vi "OutputVoltage.vi"(8 "error in":errorcluster caption="错误输入（无错误）", 9 "Channel":i32(ring)=1 items=["Channel 1"=1, "Channel 2"=2], 10 "Voltage Level":dbl format="%.3g", 11 "VISAin":refnum<visa-resource-name>) -> (0 "error out":errorcluster caption="错误输出", 1 "time":u32, 3 "VISAout":refnum<visa-resource-name>)   [LabVIEW 2013]
panel:
  out "字符串":string
  out "结果字符串":string
  in  "Current Level":dbl=0.02 format="%.3g"
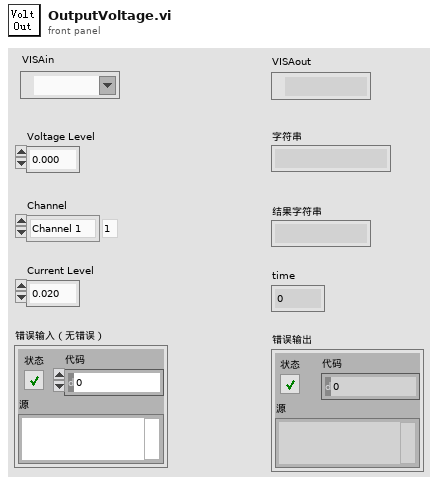
[diagram p1: front panel]
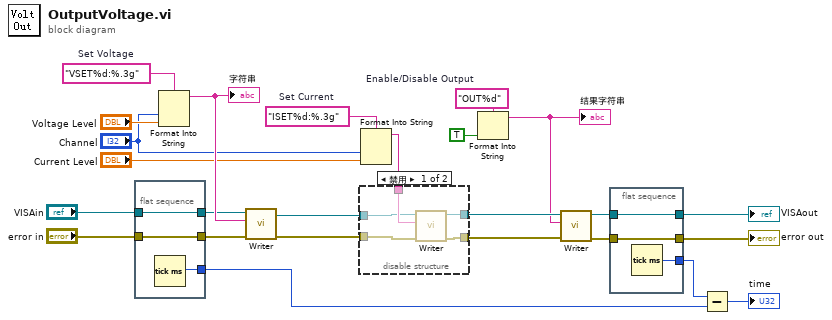
[diagram p0: block diagram]
diagram:
  w17 = "OUT%d"  # Enable/Disable Output
  w21 = "ISET%d:%.3g"  # Set Current
  w25 = "VSET%d:%.3g"  # Set Voltage
  n1 = flat-sequence {
    tunnel: "VISAin" -> [w28]
    tunnel: [w28] -> w11
    tunnel: [w27] -> w7
    tunnel: [w26] -> w5
    tunnel: "error in" -> [w26]
    frame #0 {
      n2 = Tick Count (ms)() -> (millisecond timer value=w27:u32)
    }
  }
  n3 = Format Into String(format string=w25, "Channel", "Voltage Level") -> (resulting string=w23:string)  [unwired: 2 in, 1 out]
  "字符串" <- w23
  n4 = call "Writer.vi"("error in (no error)"=w5, "Write Buffer (\"\")"=w23, "VISA resource name"=w11) -> ("error out"=w22:errorcluster, "VISA resource name out"=w18:refnum<visa-resource-name>)  [unwired: 6 in, 1 out]
  n5 = Format Into String(format string=w21, "Channel", "Current Level") -> (resulting string=w19:string)  [unwired: 2 in, 1 out]
  n6 = disable-structure shown="禁用" {
    disable-tunnel: w22 -> [w33 w34]
    disable-tunnel: w19 -> [w32 _]
    disable-tunnel: w18 -> [w31 w35]
    disable-tunnel: [w30 w34] -> w16
    disable-tunnel: [w29 w35] -> w15
    frame Disabled {
      n7 = call "Writer.vi"("error in (no error)"=w33, "Write Buffer (\"\")"=w32, "VISA resource name"=w31) -> ("error out"=w30:errorcluster, "VISA resource name out"=w29:refnum<visa-resource-name>)  [unwired: 6 in, 1 out]
    }
    frame Enabled {
    }
  }
  n8 = Format Into String(format string=w17, TRUE ("输入 1")) -> (resulting string=w14:string)  [unwired: 2 in, 1 out]
  "结果字符串" <- w14
  n9 = call "Writer.vi"("error in (no error)"=w16, "Write Buffer (\"\")"=w14, "VISA resource name"=w15) -> ("error out"=w2:errorcluster, "VISA resource name out"=w10:refnum<visa-resource-name>)  [unwired: 6 in, 1 out]
  n10 = flat-sequence {
    tunnel: w10 -> [w38]
    tunnel: [w38] -> w9
    tunnel: [w37] -> w8
    tunnel: [w36] -> w3
    tunnel: w2 -> [w36]
    frame #0 {
      n11 = Tick Count (ms)() -> (millisecond timer value=w37:u32)
    }
  }
  n12 = Subtract(x=w8, y=w7) -> (x-y=→"time":u32)
  "error out" <- w3
  "VISAout" <- w9
